vi "Launcher.vi"   [LabVIEW 2021]
uses:
  Libraries/Business Logic/Business Logic.lvlib
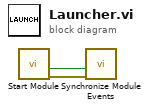
[diagram p0: block diagram]
diagram:
  n1 = call "Start Module.vi"() -> ("error out"=w2:errorcluster, "Wait for Event Sync?"=w1:bool)  [unwired: 8 in, 2 out]
  n2 = call "Synchronize Module Events.vi"("error in"=w2, "Wait for Event Sync?"=w1) -> ()  [unwired: 9 in, 1 out]
